vi "Read Image Graph.vi"(8 "error in (no error)":errorcluster, 11 "Display Image in":refnum<class "Display Image.lvclass">) -> (0 "error out":errorcluster, 2 "Image Graph":dbl[][](array[numeric]), 3 "Display Image out":refnum<class "Display Image.lvclass">)   [LabVIEW 2018, in "Display Image.lvclass"]
doc: "Este VI faz a leitura da imagem contida na classe."
uses:
  Display Image.lvclass
  Display Image.lvclass/Display Image.ctl
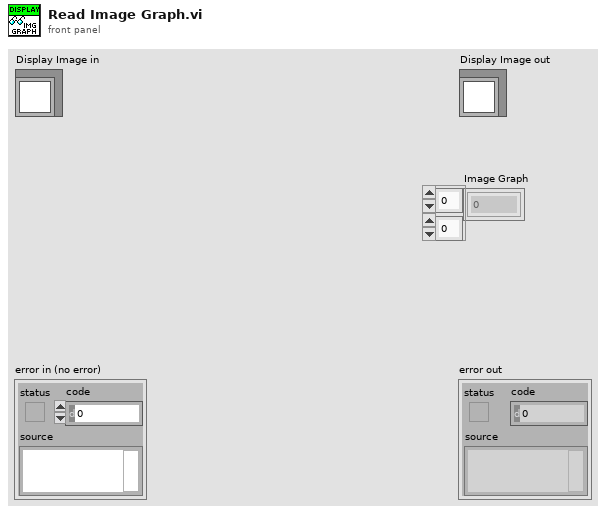
[diagram p1: front panel]
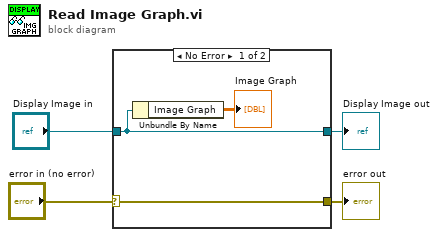
[diagram p0: block diagram]
diagram:
  n1 = case shown="No Error" "error in (no error)" {
    selector: "error in (no error)" -> [w7 w9]
    tunnel: [w7 w9] -> w3
    tunnel: [w6 w8] -> w1
    tunnel: "Display Image in" -> [w6 w8]
    frame No Error {
      n2 = Unbundle By Name(w6) -> ("Image Graph"=→"Image Graph":dbl[][])
    }
    frame Error {
    }
  }
  "error out" <- w3
  "Display Image out" <- w1
